vi "DSP Parameter Calculate.vi"(8 "error in (no error)":errorcluster caption="错误输入（无错误）", 11 "DSP Configuration":T2={"Sampling Frequency"=0.0, "filter type"=enum."Lowpass", "RF Filter Low Frequency"=0.0, "RF Filter High Frequency"=0.0, "RF Filter Taps"=0, "window"=0, "RF window parameter"=nan, "filter type 2"=enum."Lowpass", "Demodulated Filter Low Frequency"=0.0, "Demodulated Filter HighFrequency"=0.0, "Demodulated Filter Order"=0, "SPAN"=0, "Logarithmic Base"=0.0, "Noise path"="", "Work position parameter"=[]} {"window" items=["Rectangle"=0, "Hanning"=1, "Hamming"=2, "Blackman-Harris"=3, "Exact Blackman"=4, "Blackman"=5, "Flat Top"=6, "4 Term B-Harris "=7, "7 Term B-Harris"=8, "Low Sidelobe"=9, "Blackman Nuttall"=11, "Triangle"=30, "Bartlett-Hanning"=31, "Bohman"=32, "Parzen"=33, "Welch"=34, "Kaiser"=60, "Dolph-Chebyshev"=61, "Gaussian"=62]}) -> (0 "error out":errorcluster caption="错误输出", 3 "DSP Parameter":T1 {"IIR Filter Cluster"."Forward Coefficients" format="%.4f"; "IIR Filter Cluster"."Reverse Coefficients" format="%.4f"; "RF"."Forward Coefficients" format="%.4f"; "RF"."Reverse Coefficients" format="%.4f"})   [LabVIEW 2015, in "Digital Signal Processing.lvlib"]
doc: "该模板用于创建子VI。"
uses:
  Digital Signal Processing.lvlib
  Support/DSP Configuration.ctl
  <vilib>/Analysis/3filter.llb/Filter Passband Type.ctl
  <vilib>/Analysis/4window.llb/windowTd.ctl
  Support/DSP Parameter.ctl
  <vilib>/Analysis/NI_AALBase.lvlib
  <vilib>/Analysis/NI_AALPro.lvlib
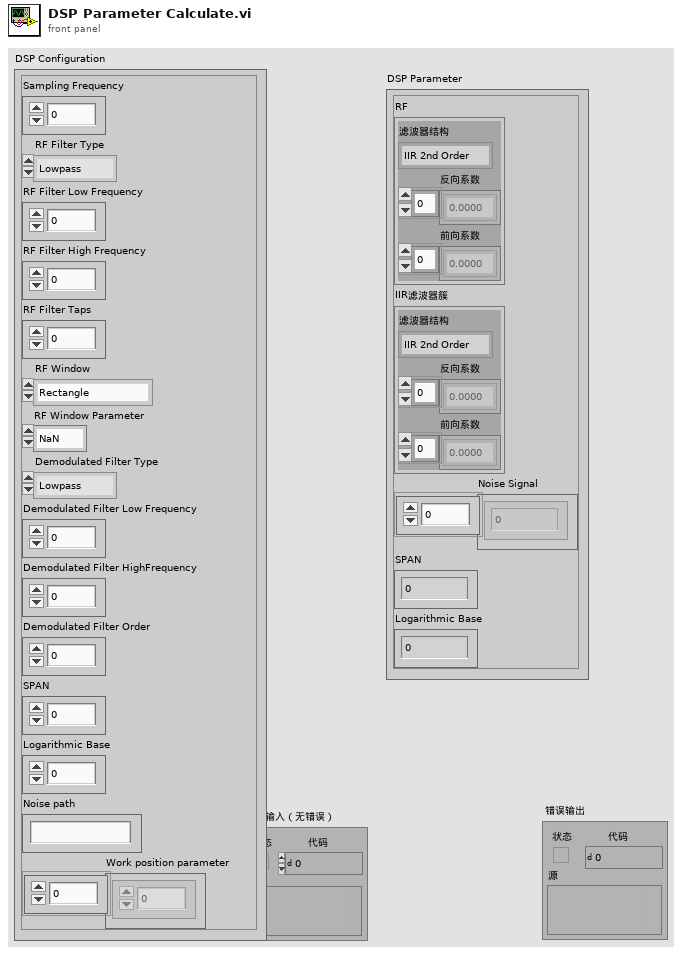
[diagram p1: front panel]
types:
  T1 = typedef "Digital Signal Processing.lvlib/DSP Parameter.ctl" = cluster{"RF":cluster{"filter structure":enum32{"IIR 2nd Order", "IIR 4th Order"}, "Reverse Coefficients":dbl[], "Forward Coefficients":dbl[]}, "IIR Filter Cluster":cluster{"filter structure":enum32{"IIR 2nd Order", "IIR 4th Order"}, "Reverse Coefficients":dbl[], "Forward Coefficients":dbl[]}, "Noise Signal":dbl[], "SPAN":i32, "Logarithmic Base":dbl}
  T2 = typedef "Digital Signal Processing.lvlib/DSP Configuration.ctl" = cluster{"Sampling Frequency":dbl, "filter type":T3, "RF Filter Low Frequency":dbl, "RF Filter High Frequency":dbl, "RF Filter Taps":i32, "window":T4, "RF window parameter":dbl, "filter type 2":T3, "Demodulated Filter Low Frequency":dbl, "Demodulated Filter HighFrequency":dbl, "Demodulated Filter Order":i32, "SPAN":i32, "Logarithmic Base":dbl, "Noise path":string, "Work position parameter":i32[]}
  T3 = typedef "NI_AALBase.lvlib/Filter Passband Type.ctl" = enum32{"Lowpass", "Highpass", "Bandpass", "Bandstop"}
  T4 = typedef "NI_AALPro.lvlib/windowTd.ctl" = u32
  T5 = cluster{"filter structure":enum32{"IIR 2nd Order", "IIR 4th Order"}, "Reverse Coefficients":dbl[], "Forward Coefficients":dbl[]}
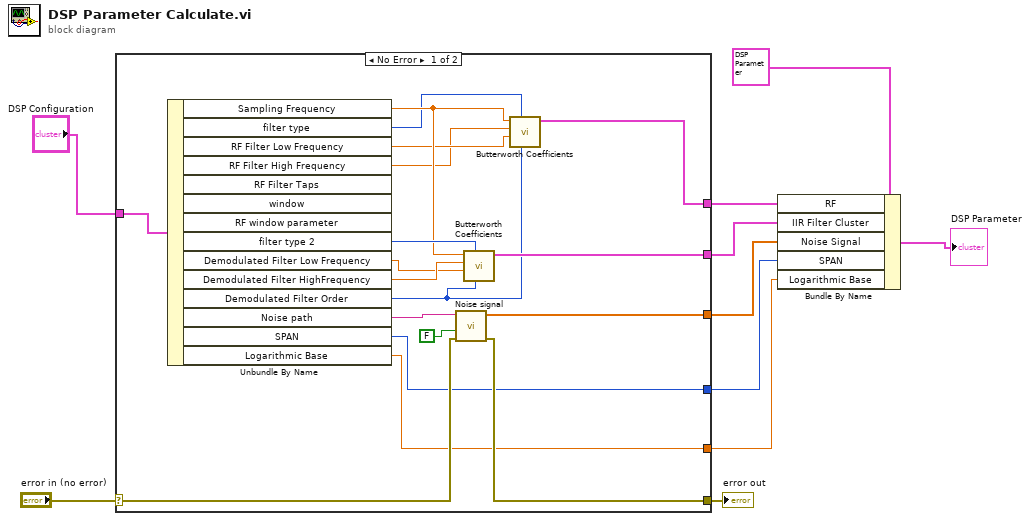
[diagram p0: block diagram]
diagram:
  n1 = case shown="No Error" "error in (no error)" {
    selector: "error in (no error)" -> [w20 w29]
    tunnel: [w19 w29] -> w9
    tunnel: "DSP Configuration" -> [w23 _]
    tunnel: [w22 _] -> w6
    tunnel: [w21 _] -> w5
    tunnel: [w18 _] -> w4
    tunnel: [w17 _] -> w3
    tunnel: [w11 _] -> w1
    frame No Error {
      n2 = Unbundle By Name(w23) -> ("Sampling Frequency"=w16:dbl, "filter type"=w13:T3, "RF Filter Low Frequency"=w15:dbl, "RF Filter High Frequency"=w14:dbl, "filter type 2"=w26:T3, "Demodulated Filter Low Frequency"=w24:dbl, "Demodulated Filter HighFrequency"=w25:dbl, "Demodulated Filter Order"=w12:i32, "Noise path"=w28:string, "SPAN"=w18:i32, "Logarithmic Base"=w17:dbl)  [unwired: 3 out]
      n3 = call "Noise signal.vi"("错误输入"=w20, "写入（非为读取）"=FALSE, "Path"=w28) -> ("错误输出"=w19:errorcluster, "output signal"=w21:dbl[])  [unwired: 7 in]
      n4 = call <vilib>:"Butterworth Coefficients.vi"("order"=w12, "filter type"=w26, "low cutoff freq: fl"=w24, "high cutoff freq: fh"=w25, "sampling freq: fs"=w16) -> ("IIR Filter Cluster"=w22:T5)  [unwired: 5 in, 1 out]
      n5 = call <vilib>:"Butterworth Coefficients.vi"("order"=w12, "filter type"=w13, "low cutoff freq: fl"=w15, "high cutoff freq: fh"=w14, "sampling freq: fs"=w16) -> ("IIR Filter Cluster"=w11:T5)  [unwired: 5 in, 1 out]
    }
    frame Error {
    }
  }
  "error out" <- w9
  n6 = Bundle By Name(cluster=T1 {"RF"={"filter structure"=enum."IIR 2nd Order", "Reverse Coefficients"=[], "Forward Coefficients"=[]}, "IIR Filter Cluster"={"filter structure"=enum."IIR 2nd Order", "Reverse Coefficients"=[], "Forward Coefficients"=[]}, "Noise Signal"=[], "SPAN"=0, "Logarithmic Base"=0.0} ("DSP Parameter"), "RF"=w1, "IIR Filter Cluster"=w6, "Noise Signal"=w5, "SPAN"=w4, "Logarithmic Base"=w3) -> (→"DSP Parameter":T1)
